vi "Set Window Position.vi"(9 "Ctl Refnum":refnum<vi>, 11 "VI in":refnum<vi>) -> (3 "VI out":refnum<vi>)   [LabVIEW 2020]
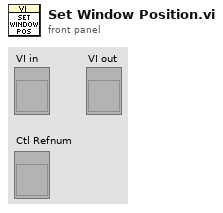
[diagram p1: front panel]
types:
  T1 = typedef "LVRectTypeDef.ctl" = cluster{"Left":i16, "Top":i16, "Right":i16, "Bottom":i16}
  T2 = cluster{"Left":i16, "Top":i16, "Right":i16, "Bottom":i16, "Width":i16, "Height":i16}
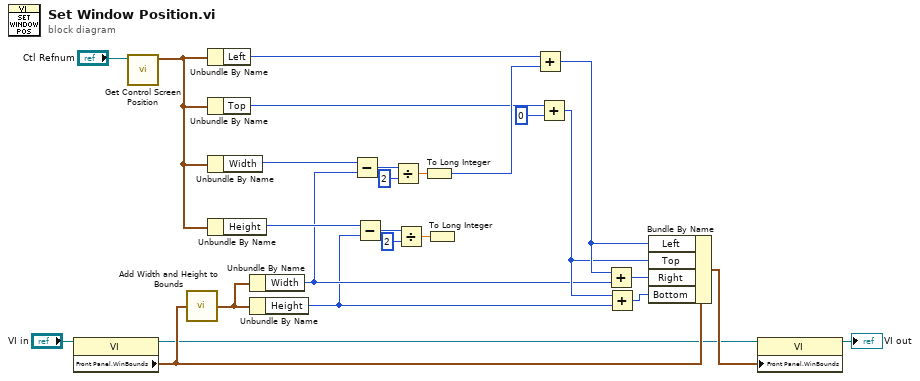
[diagram p0: block diagram]
diagram:
  n1 = property class="VI"(reference="VI in") -> (reference out=w8:refnum<vi>, "Front Panel.WinBounds"=w16:T1)  [unwired: 1 in, 1 out]
  n2 = call "Get Control Screen Position.vi"("Control in"="Ctl Refnum") -> ("Bounds Out"=w5:T2)  [unwired: 10 in]
  n3 = call "Add Width and Height to Bounds.vi"("WinBounds"=w16) -> ("Bounds Out"=w17:T2)
  n4 = Unbundle By Name(w5) -> ("Left"=w6:i16)
  n5 = Unbundle By Name(w5) -> ("Top"=w4:i16)
  n6 = Unbundle By Name(w5) -> ("Width"=w26:i16)
  n7 = Unbundle By Name(w5) -> ("Height"=w21:i16)
  n8 = Unbundle By Name(w17) -> ("Width"=w11:i16)
  n9 = Unbundle By Name(w17) -> ("Height"=w10:i16)
  n10 = Subtract(x=w26, y=w11) -> (x-y=w25:i16)
  n11 = Subtract(x=w21, y=w10) -> (x-y=w20:i16)
  n12 = Divide(x=w25, y=u32 2) -> (x/y=w23:dbl)
  n13 = Divide(x=w20, y=u32 2) -> (x/y=w18:dbl)
  n14 = To Long Integer(number=w23) -> (32bit integer=w22:i32)
  n15 = To Long Integer(number=w18) -> ()  [unwired: 1 out]
  n16 = Add(x=w6, y=w22) -> (x+y=w14:i32)
  n17 = Add(x=w4, y=i16 0) -> (x+y=w12:i16)
  n18 = Add(x=w14, y=w11) -> (x+y=w15:i32)
  n19 = Add(x=w12, y=w10) -> (x+y=w13:i16)
  n20 = Bundle By Name(cluster=w16, "Left"=w14, "Top"=w12, "Right"=w15, "Bottom"=w13) -> (w9:T1)
  n21 = property class="VI"(reference=w8, "Front Panel.WinBounds"=w9) -> (reference out=→"VI out":refnum<vi>)  [unwired: 1 in, 1 out]
